vi "ObjectTrackingOld.vi"(7 "error in":errorcluster) -> (0 "error out":errorcluster, 1 "Frame Rate":dbl, 2 "Location.Y":dbl(slide) scale=0.0..240.0, 3 "Location.X":dbl(slide) scale=0.0..320.0, 4 "Image Out":T2(plugin-control))   [LabVIEW 2016]
panel:
  out "Fitted Circle (Find Circular Edge 1)":T1 {"Average SNR (dB)" format="%.2f"; "Average Strength" format="%.2f"; "Roundness (Real-World)" format="%.2f"; "Radius (Real-World)" format="%.2f"; "Center (Real-World)"."Y" format="%.2f"; "Center (Real-World)"."X" format="%.2f"; "Radius (Pixels)" format="%.2f"; "Center (Pixels)"."Y" format="%.2f"; "Center (Pixels)"."X" format="%.2f"}
  in  "Stop (F)":bool
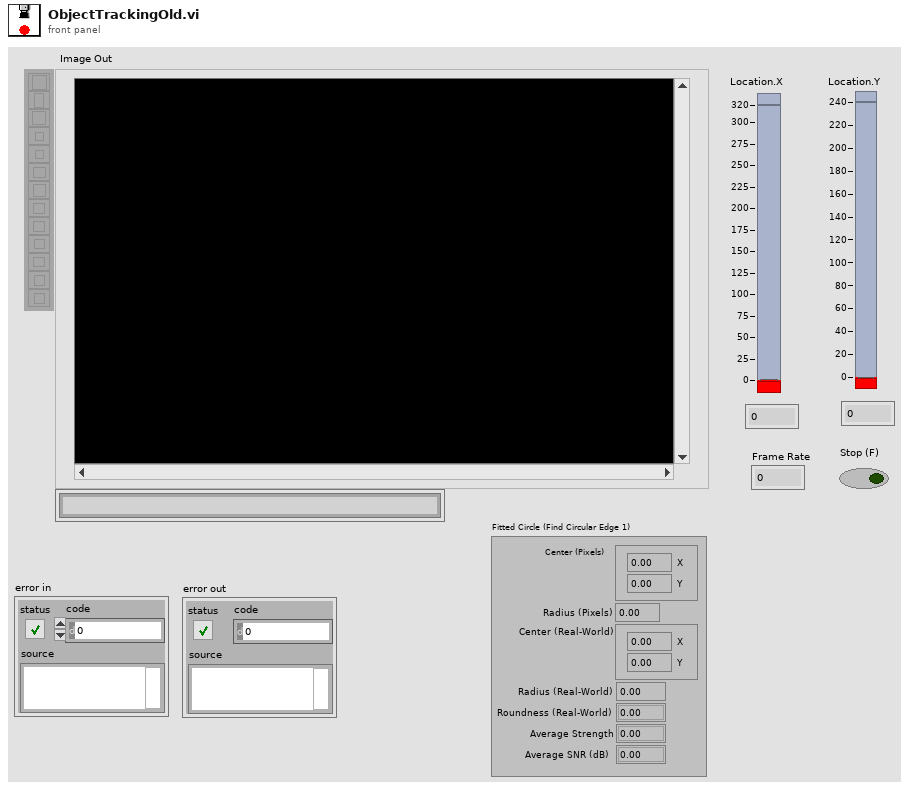
[diagram p1: front panel]
types:
  T1 = cluster{"Center (Pixels)":cluster{"X":sgl, "Y":sgl}, "Radius (Pixels)":dbl, "Center (Real-World)":cluster{"X":sgl, "Y":sgl}, "Radius (Real-World)":dbl, "Roundness (Real-World)":dbl, "Average Strength":dbl, "Average SNR (dB)":dbl}
  T2 = typedef "IMAQ Image.ctl" = refnum<image>
  T3 = cluster{"Label":string, "Score":i32, "Angle":dbl, "Location":cluster{"X":dbl, "Y":dbl}, "Bounding Box":cluster{"X":dbl, "Y":dbl}[], "Object Found?":bool}[]
  T4 = cluster{"Label":string, "Score":i32, "Angle":dbl, "Location":cluster{"X":dbl, "Y":dbl}, "Bounding Box":cluster{"X":dbl, "Y":dbl}[], "Object Found?":bool}
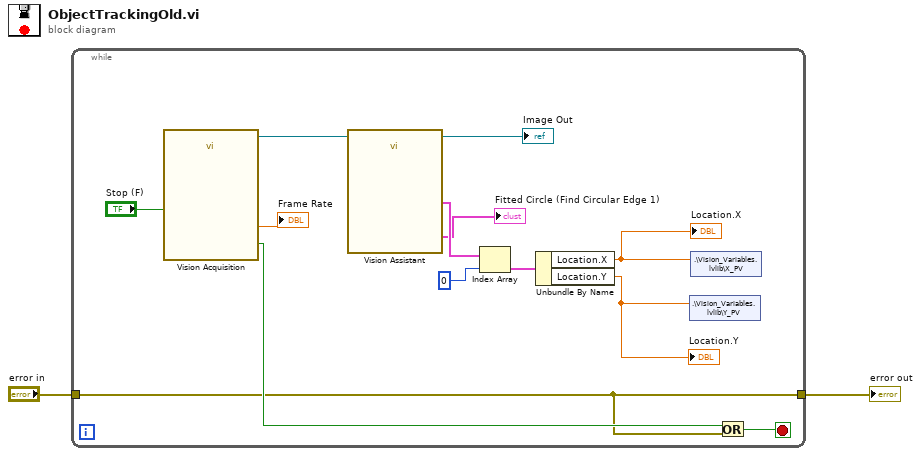
[diagram p0: block diagram]
diagram:
  n1 = while {
    tunnel: "error in" -> [w5]
    tunnel: [w5] -> w1
    stop <- w6 stop-if-true
    n2 = call "Vision Acquisition"("Stop (F)"="Stop (F)") -> ("Image Out"=w11:T2, "Frame Rate"=→"Frame Rate":dbl, "Stopped"=w12:bool)  [unwired: 23 in, 1 out]
    n3 = call "Vision Assistant"("Image In"=w11) -> ("Image Out"=→"Image Out":T2, "Objects (pixel) (Object Tracking 1)"=w9:T3, "Fitted Circle (Find Circular Edge 1)"=→"Fitted Circle (Find Circular Edge 1)":T1)  [unwired: 22 in, 2 out]
    n4 = Index Array(array=w9, index=0) -> (element=w8:T4)
    n5 = Unbundle By Name(w8) -> ("Location.X"=w4:dbl, "Location.Y"=w3:dbl)
    "Location.X" <- w4
    "Location.Y" <- w3
    n6 = shared-variable ".\\Vision_Variables.lvlib\\Y_PV"(w3) -> ()  [unwired: 1 in, 1 out]
    n7 = shared-variable ".\\Vision_Variables.lvlib\\X_PV"(w4) -> ()  [unwired: 1 in, 1 out]
    n8 = Or(x=w12, y=w5) -> (x .or. y?=w6:bool)
  }
  "error out" <- w1
